vi "divert beam.vi"(7 "divert beam?":u16(ring) items=["allow beam", "divert beam"], 8 "error in":errorcluster, 11 "task/channels in":refnum<k21>) -> (0 "error out":errorcluster, 3 "task out":refnum<k21>)   [LabVIEW 2016]
doc: "creates or a high or low( divert or accept) digital signal"
uses:
  <vilib>/DAQmx/write.llb/DAQmx Write (Digital Wfm 1Chan NSamp).vi
  <vilib>/Waveform/DWDTOps.llb/DWDT Boolean Array to Digital.vi
  <vilib>/DAQmx/configure/timing.llb/DAQmx Timing (Burst Import Clock).vi
  <vilib>/Waveform/DWDTOps.llb/DWDT Uncompress Digital.vi
  <vilib>/DAQmx/miscellaneous.llb/DAQmx Fill In Error Info.vi
  <resource>/objmgr/daqmx.rc
panel:
  out "error out 3":errorcluster
  out "error out 6":errorcluster
  out "error out 2":errorcluster
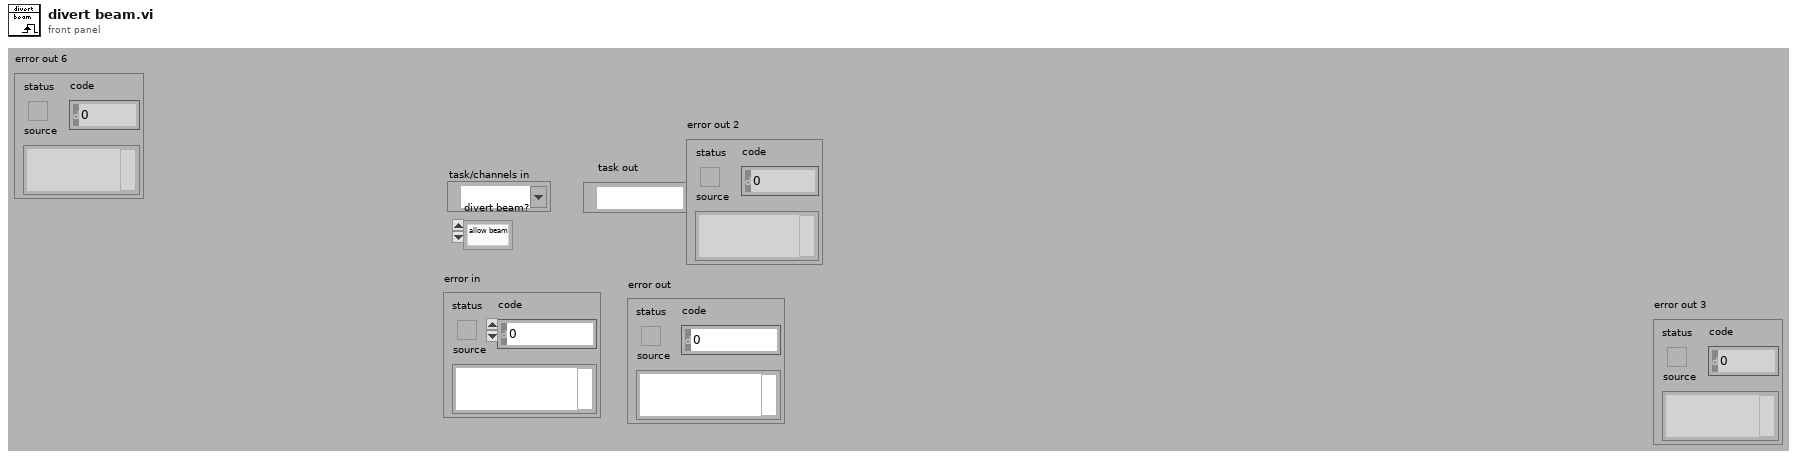
[diagram p1: front panel]
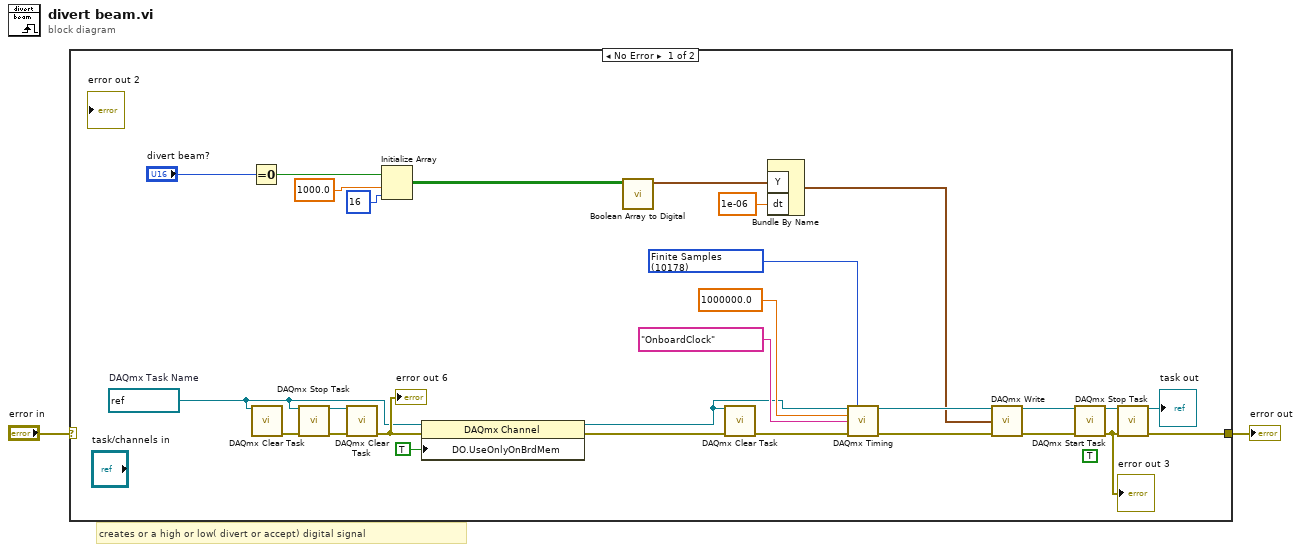
[diagram p0: block diagram]
diagram:
  # "creates or a high or low( divert or accept) digital signal"
  n1 = case shown="No Error" "error in" {
    selector: "error in" -> [_ w31]
    tunnel: [w4 w31] -> w1
    frame No Error {
      w3 = refnum<k21> "chop2"  # DAQmx Task Name
      w25 = 10178 items=["Finite Samples"=10178, "Continuous Samples"=10123, "Hardware Timed Single Point"=12522] ("sample mode")
      (unwired) TRUE ("auto start")
      n2 = Equal To 0?(x="divert beam?") -> (x = 0?=w5:bool)
      n3 = call <vilib>:"DAQmx Clear Task.vi"("task in"=w3) -> ("error out"=w10:errorcluster)  [unwired: 14 in]
      n4 = call <vilib>:"DAQmx Stop Task.vi"("task/channels in"=w3, "error in"=w10) -> ("task out"=w19:refnum<k21>, "error out"=w21:errorcluster)  [unwired: 12 in]
      n5 = call <vilib>:"DAQmx Clear Task.vi"("task in"=w19, "error in"=w21) -> ("error out"=w22:errorcluster)  [unwired: 13 in]
      "error out 6" <- w22
      n6 = Initialize Array(w5, 1000.0 ("x"), 16 ("dimension size")) -> (w28:bool[][])
      n7 = property class="DAQmx Channel"(reference=w3, error in=w22, "DO.UseOnlyOnBrdMem"=TRUE) -> (reference out=w12:refnum<k21>, error out=w16:errorcluster)
      n8 = call-poly <vilib>:"Boolean Array to Digital.vi"("boolean array"=w28) -> ("digital waveform"=w27:digitalwaveform)  [unwired: 9 in, 1 out]
      n9 = call <vilib>:"DAQmx Clear Task.vi"("task in"=w12, "error in"=w16) -> ("error out"=w15:errorcluster)  [unwired: 13 in]
      n10 = Bundle By Name("Y"=w27, "dt"=1e-06) -> (w11:digitalwaveform)  [unwired: 1 in]
      n11 = call-poly <vilib>:"DAQmx Timing.vi"("task/channels in"=w12, "sample mode"=w25, "sample clock rate"=1000000.0 ("rate"), "sample clock source"=tag "OnboardClock", "error in"=w15) -> ("task out"=w17:refnum<k21>, "error out"=w18:errorcluster)  [unwired: 9 in]
      n12 = call-poly <vilib>:"DAQmx Write.vi"("task/channels in"=w17, "data"=w11, "error in"=w18) -> ("task out"=w24:refnum<k21>, "error out"=w23:errorcluster)  [unwired: 10 in, 1 out]
      n13 = call <vilib>:"DAQmx Start Task.vi"("task/channels in"=w24, "error in"=w23) -> ("task out"=w9:refnum<k21>, "error out"=w8:errorcluster)  [unwired: 12 in]
      "error out 3" <- w8
      n14 = call <vilib>:"DAQmx Stop Task.vi"("task/channels in"=w9, "error in"=w8) -> ("task out"=→"task out":refnum<k21>, "error out"=w4:errorcluster)  [unwired: 12 in]
    }
    frame Error {
    }
  }
  "error out" <- w1
